vi "Physics_Model.vi"() -> ()   [LabVIEW 2025]
panel:
  out "RPM":dbl
  out "Speed_New":dbl
  in  "Tilt_sensor":dbl
  in  "Brake[%]":dbl
  in  "Throttle[%]":dbl
  in  "Prev_Speed[km/h]":dbl
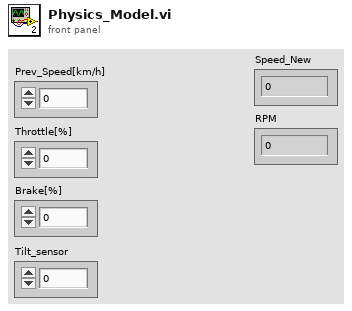
[diagram p1: front panel]
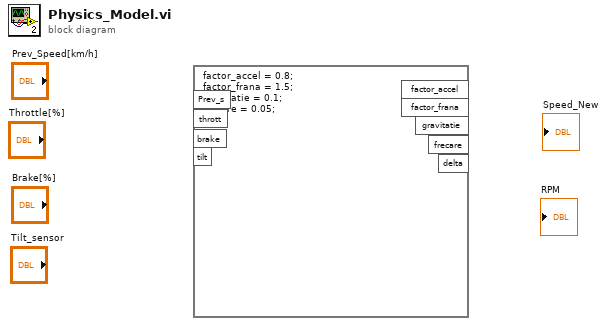
[diagram p0: block diagram]
diagram:
  n1 = formula code="factor_accel = 0.8;\nfactor_frana = 1.5;\ngravitatie = 0.1;\nfrecare = 0.05;\ndelta"() -> ()  [unwired: 1 in, 8 out]
